vi "GFITS_WriteFileMsg.vi"(4 "status":string, 6 "expID":string, 8 "error in":errorcluster, 9 "image name (no ext)":string, 10 "filemsg":string, 11 "Database RefNum":T1) -> ()   [LabVIEW 2016]
uses:
  DBSHAND/private/vis/DatabaseHand_RefNum.ctl
  DBSHAND/private/vis/DatabaseHand_Element_Get(string).vi
panel:
  out "error out":errorcluster
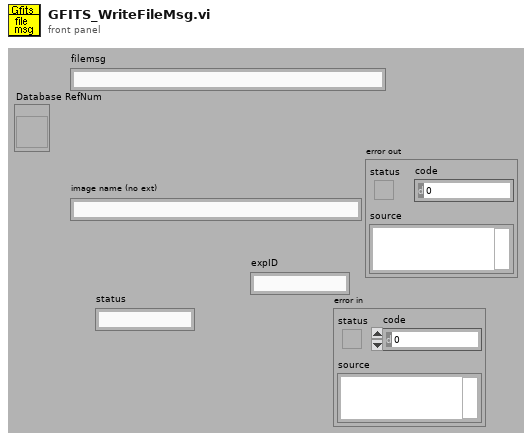
[diagram p1: front panel]
types:
  T1 = typedef "DatabaseHand_RefNum.ctl" = refnum<vi>
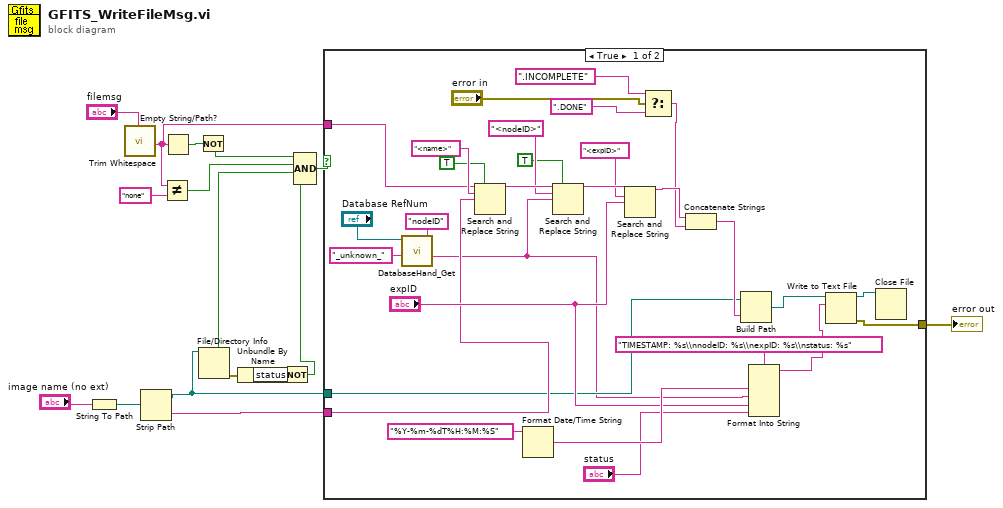
[diagram p0: block diagram]
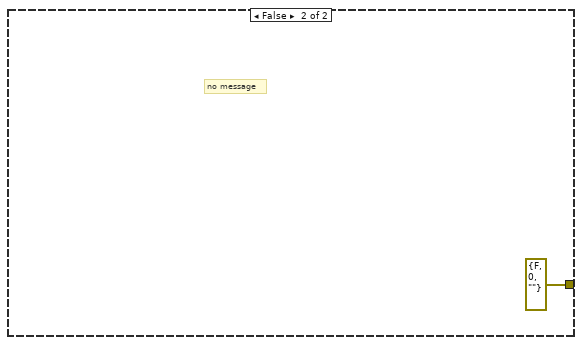
[diagram p2: hidden frame]
diagram:
  n1 = String To Path(string="image name (no ext)") -> (path=w11:path)
  n2 = call <vilib>:"Trim Whitespace.vi"("string"="filemsg") -> ("trimmed string"=w5:string)  [unwired: 1 in]
  n3 = Strip Path(path=w11) -> (stripped path=w8:path, name=w9:string)
  n4 = Not Equal?(x=w5, y="none") -> (x != y?=w3:bool)
  n5 = Empty String/Path?(string/path=w5) -> (empty?=w14:bool)
  n6 = Not(x=w14) -> (.not. x?=w13:bool)
  n7 = File/Directory Info(path=w8) -> (directory=w2:bool, error out=w7:errorcluster)  [unwired: 1 in, 5 out]
  n8 = Unbundle By Name(w7) -> ("status"=w6:bool)
  n9 = Not(x=w6) -> (.not. x?=w1:bool)
  n10 = Compound Arithmetic op=AND(w13, w3, w2, w1) -> (w12:bool)
  n11 = case shown="True" w12 {
    tunnel: [w34 errorcluster {"status"=FALSE, "code"=0, "source"=""} ("error out")] -> w15
    tunnel: w5 -> [w28 _]
    tunnel: w9 -> [w27 _]
    tunnel: w8 -> [w26 _]
    frame True {
      n12 = call-poly "DatabaseHand_Get.vi"("default value"="_unknown_", "name"="nodeID", "Database RefNum in"="Database RefNum") -> ("value"=w23:string)  [unwired: 2 in, 6 out]
      n13 = Search and Replace String(replace all?=TRUE ("replace all? (F)"), input string=w28, search string="<name>" ("regular expression"), replace string=w27) -> (result string=w44:string)  [unwired: 1 in, 6 out]
      n14 = Format Date/Time String(time format string (%c)="%Y-%m-%dT%H:%M:%S") -> (date/time string=w32:string)  [unwired: 2 out]
      n15 = Search and Replace String(replace all?=TRUE ("replace all? (F)"), input string=w44, search string="<nodeID>", replace string=w23) -> (result string=w40:string)  [unwired: 1 in, 6 out]
      n16 = Search and Replace String(input string=w40, search string="<expID>", replace string="expID") -> (result string=w38:string)  [unwired: 1 in, 7 out]
      n17 = Select(t=".INCOMPLETE" ("string"), s="error in", f=".DONE" ("string")) -> (s? t:f=w18:string)
      n18 = Concatenate Strings(w38, w18) -> (w37:string)
      n19 = Build Path(base path=w26, name or relative path=w37) -> (appended path=w36:path)
      n20 = Format Into String(format string="TIMESTAMP: %s\\nnodeID: %s\\nexpID: %s\\nstatus: %s", w32, w23, "expID", "status") -> (resulting string=w31:string)  [unwired: 2 in, 1 out]
      n21 = Write to Text File(file (use dialog)=w36, text=w31) -> (refnum out=w17:refnum<file>, error out=w34:errorcluster)  [unwired: 1 in, 2 out]
      n22 = Close File(refnum=w17) -> ()  [unwired: 1 in, 2 out]
    }
    frame False {
      # "no message"
    }
  }
  "error out" <- w15
